vi "JT_Set_Monitor_Values.vi"(2 "Plot-Control":T1={"V2"=FALSE, "V5"=FALSE, "V1"=FALSE, "V9"=TRUE, "F"=TRUE, "C"=FALSE, "V4"=FALSE, "Dump"=0, "P3"=0.0, "P1"=0.0, "P2"=0.0, "P5"=18.434412358753207, "Box Temp"=18.434412358753207, "Pressure 1"=0, "Pressure 2"=0, "Pressure 3"=15, "Pressure 4"=13, "Setpoint"=0.0, "MC Heater Output"=0.0, "Still Heater Output"=0.0, "Sorb  Heater Output"=0.0, "Heater"=[], "Pressures"=[]} {"Pressure 4" items=["Time", "LI1CH1", "LI1CH2", "LI2CH1", "LI2CH2", "LI3CH1", "LI3CH2", "Field", "Temperature", "Temperature 2", "Temperatrue 3", "Nitrogen_Level", "Helium_Level", "Heater_LS370", "Sorb_Heater", "Still_Heater", "Capacity", "Loss", "Magnet_Temperature", "Lambda_Pressure", "Lambda_Needle_Valve", "LS370-CH1-T", "LS370-CH2-T", "LS370-CH3-T", "LS370-CH4-T", "LS370-TC-T", "LS370-CH1-R", "LS370-CH2-R", "LS370-CH3-R", "LS370-CH4-R", "LS370-TC-R", "LS372-CH1-T", "LS372-CH2-T", "LS372-CH3-T", "LS372-CH4-T", "LS372-CH5-T", "LS372-CH1-R", "LS372-CH2-R", "LS372-CH3-R", "LS372-CH4-R", "LS372-CH5-R", "Nada", "Keithley_Res", "Keithley_Current", "VTI_Heater", "VTI_Needle Valve", "LS340_Heater", "Keithley_6221_Amplitude", "Keithley_6221_Frequency", "Condense_Pressure", "Still_Pressure", "FP_Out_Pressure", "Dump_Pressure", "V1", "V2", "V4", "V5", "V9", "Forepump", "Compressor", "Keihtley_6221_Offset", "BoxTemp", "By", "Bz", "Phi", "heater-recond (%)", "Dewar Pressure "]; "Pressure 3" items=["Time", "LI1CH1", "LI1CH2", "LI2CH1", "LI2CH2", "LI3CH1", "LI3CH2", "Field", "Temperature", "Temperature 2", "Temperatrue 3", "Nitrogen_Level", "Helium_Level", "Heater_LS370", "Sorb_Heater", "Still_Heater", "Capacity", "Loss", "Magnet_Temperature", "Lambda_Pressure", "Lambda_Needle_Valve", "LS370-CH1-T", "LS370-CH2-T", "LS370-CH3-T", "LS370-CH4-T", "LS370-TC-T", "LS370-CH1-R", "LS370-CH2-R", "LS370-CH3-R", "LS370-CH4-R", "LS370-TC-R", "LS372-CH1-T", "LS372-CH2-T", "LS372-CH3-T", "LS372-CH4-T", "LS372-CH5-T", "LS372-CH1-R", "LS372-CH2-R", "LS372-CH3-R", "LS372-CH4-R", "LS372-CH5-R", "Nada", "Keithley_Res", "Keithley_Current", "VTI_Heater", "VTI_Needle Valve", "LS340_Heater", "Keithley_6221_Amplitude", "Keithley_6221_Frequency", "Condense_Pressure", "Still_Pressure", "FP_Out_Pressure", "Dump_Pressure", "V1", "V2", "V4", "V5", "V9", "Forepump", "Compressor", "Keihtley_6221_Offset", "BoxTemp", "By", "Bz", "Phi", "heater-recond (%)", "Dewar Pressure "]; "Pressure 2" items=["Time", "LI1CH1", "LI1CH2", "LI2CH1", "LI2CH2", "LI3CH1", "LI3CH2", "Field", "Temperature", "Temperature 2", "Temperatrue 3", "Nitrogen_Level", "Helium_Level", "Heater_LS370", "Sorb_Heater", "Still_Heater", "Capacity", "Loss", "Magnet_Temperature", "Lambda_Pressure", "Lambda_Needle_Valve", "LS370-CH1-T", "LS370-CH2-T", "LS370-CH3-T", "LS370-CH4-T", "LS370-TC-T", "LS370-CH1-R", "LS370-CH2-R", "LS370-CH3-R", "LS370-CH4-R", "LS370-TC-R", "LS372-CH1-T", "LS372-CH2-T", "LS372-CH3-T", "LS372-CH4-T", "LS372-CH5-T", "LS372-CH1-R", "LS372-CH2-R", "LS372-CH3-R", "LS372-CH4-R", "LS372-CH5-R", "Nada", "Keithley_Res", "Keithley_Current", "VTI_Heater", "VTI_Needle Valve", "LS340_Heater", "Keithley_6221_Amplitude", "Keithley_6221_Frequency", "Condense_Pressure", "Still_Pressure", "FP_Out_Pressure", "Dump_Pressure", "V1", "V2", "V4", "V5", "V9", "Forepump", "Compressor", "Keihtley_6221_Offset", "BoxTemp", "By", "Bz", "Phi", "heater-recond (%)", "Dewar Pressure "]; "Pressure 1" items=["Time", "LI1CH1", "LI1CH2", "LI2CH1", "LI2CH2", "LI3CH1", "LI3CH2", "Field", "Temperature", "Temperature 2", "Temperatrue 3", "Nitrogen_Level", "Helium_Level", "Heater_LS370", "Sorb_Heater", "Still_Heater", "Capacity", "Loss", "Magnet_Temperature", "Lambda_Pressure", "Lambda_Needle_Valve", "LS370-CH1-T", "LS370-CH2-T", "LS370-CH3-T", "LS370-CH4-T", "LS370-TC-T", "LS370-CH1-R", "LS370-CH2-R", "LS370-CH3-R", "LS370-CH4-R", "LS370-TC-R", "LS372-CH1-T", "LS372-CH2-T", "LS372-CH3-T", "LS372-CH4-T", "LS372-CH5-T", "LS372-CH1-R", "LS372-CH2-R", "LS372-CH3-R", "LS372-CH4-R", "LS372-CH5-R", "Nada", "Keithley_Res", "Keithley_Current", "VTI_Heater", "VTI_Needle Valve", "LS340_Heater", "Keithley_6221_Amplitude", "Keithley_6221_Frequency", "Condense_Pressure", "Still_Pressure", "FP_Out_Pressure", "Dump_Pressure", "V1", "V2", "V4", "V5", "V9", "Forepump", "Compressor", "Keihtley_6221_Offset", "BoxTemp", "By", "Bz", "Phi", "heater-recond (%)", "Dewar Pressure "]; "Dump" scale=0.0..100.0}, 3 "X-Axis (S)":i32, 4 "Measurement Time (s)":dbl format="%#_13g", 5 "System Monitor Variables (in)":T2) -> (0 "Cluster":T1={"V2"=FALSE, "V5"=FALSE, "V1"=FALSE, "V9"=TRUE, "F"=TRUE, "C"=FALSE, "V4"=FALSE, "Dump"=0, "P3"=0.0, "P1"=0.0, "P2"=0.0, "P5"=18.434412358753207, "Box Temp"=18.434412358753207, "Pressure 1"=0, "Pressure 2"=0, "Pressure 3"=15, "Pressure 4"=13, "Setpoint"=0.0, "MC Heater Output"=0.0, "Still Heater Output"=0.0, "Sorb  Heater Output"=0.0, "Heater"=[], "Pressures"=[]} {"Pressure 4" items=["Time", "LI1CH1", "LI1CH2", "LI2CH1", "LI2CH2", "LI3CH1", "LI3CH2", "Field", "Temperature", "Temperature 2", "Temperatrue 3", "Nitrogen_Level", "Helium_Level", "Heater_LS370", "Sorb_Heater", "Still_Heater", "Capacity", "Loss", "Magnet_Temperature", "Lambda_Pressure", "Lambda_Needle_Valve", "LS370-CH1-T", "LS370-CH2-T", "LS370-CH3-T", "LS370-CH4-T", "LS370-TC-T", "LS370-CH1-R", "LS370-CH2-R", "LS370-CH3-R", "LS370-CH4-R", "LS370-TC-R", "LS372-CH1-T", "LS372-CH2-T", "LS372-CH3-T", "LS372-CH4-T", "LS372-CH5-T", "LS372-CH1-R", "LS372-CH2-R", "LS372-CH3-R", "LS372-CH4-R", "LS372-CH5-R", "Nada", "Keithley_Res", "Keithley_Current", "VTI_Heater", "VTI_Needle Valve", "LS340_Heater", "Keithley_6221_Amplitude", "Keithley_6221_Frequency", "Condense_Pressure", "Still_Pressure", "FP_Out_Pressure", "Dump_Pressure", "V1", "V2", "V4", "V5", "V9", "Forepump", "Compressor", "Keihtley_6221_Offset", "BoxTemp", "By", "Bz", "Phi", "heater-recond (%)", "Dewar Pressure "]; "Pressure 3" items=["Time", "LI1CH1", "LI1CH2", "LI2CH1", "LI2CH2", "LI3CH1", "LI3CH2", "Field", "Temperature", "Temperature 2", "Temperatrue 3", "Nitrogen_Level", "Helium_Level", "Heater_LS370", "Sorb_Heater", "Still_Heater", "Capacity", "Loss", "Magnet_Temperature", "Lambda_Pressure", "Lambda_Needle_Valve", "LS370-CH1-T", "LS370-CH2-T", "LS370-CH3-T", "LS370-CH4-T", "LS370-TC-T", "LS370-CH1-R", "LS370-CH2-R", "LS370-CH3-R", "LS370-CH4-R", "LS370-TC-R", "LS372-CH1-T", "LS372-CH2-T", "LS372-CH3-T", "LS372-CH4-T", "LS372-CH5-T", "LS372-CH1-R", "LS372-CH2-R", "LS372-CH3-R", "LS372-CH4-R", "LS372-CH5-R", "Nada", "Keithley_Res", "Keithley_Current", "VTI_Heater", "VTI_Needle Valve", "LS340_Heater", "Keithley_6221_Amplitude", "Keithley_6221_Frequency", "Condense_Pressure", "Still_Pressure", "FP_Out_Pressure", "Dump_Pressure", "V1", "V2", "V4", "V5", "V9", "Forepump", "Compressor", "Keihtley_6221_Offset", "BoxTemp", "By", "Bz", "Phi", "heater-recond (%)", "Dewar Pressure "]; "Pressure 2" items=["Time", "LI1CH1", "LI1CH2", "LI2CH1", "LI2CH2", "LI3CH1", "LI3CH2", "Field", "Temperature", "Temperature 2", "Temperatrue 3", "Nitrogen_Level", "Helium_Level", "Heater_LS370", "Sorb_Heater", "Still_Heater", "Capacity", "Loss", "Magnet_Temperature", "Lambda_Pressure", "Lambda_Needle_Valve", "LS370-CH1-T", "LS370-CH2-T", "LS370-CH3-T", "LS370-CH4-T", "LS370-TC-T", "LS370-CH1-R", "LS370-CH2-R", "LS370-CH3-R", "LS370-CH4-R", "LS370-TC-R", "LS372-CH1-T", "LS372-CH2-T", "LS372-CH3-T", "LS372-CH4-T", "LS372-CH5-T", "LS372-CH1-R", "LS372-CH2-R", "LS372-CH3-R", "LS372-CH4-R", "LS372-CH5-R", "Nada", "Keithley_Res", "Keithley_Current", "VTI_Heater", "VTI_Needle Valve", "LS340_Heater", "Keithley_6221_Amplitude", "Keithley_6221_Frequency", "Condense_Pressure", "Still_Pressure", "FP_Out_Pressure", "Dump_Pressure", "V1", "V2", "V4", "V5", "V9", "Forepump", "Compressor", "Keihtley_6221_Offset", "BoxTemp", "By", "Bz", "Phi", "heater-recond (%)", "Dewar Pressure "]; "Pressure 1" items=["Time", "LI1CH1", "LI1CH2", "LI2CH1", "LI2CH2", "LI3CH1", "LI3CH2", "Field", "Temperature", "Temperature 2", "Temperatrue 3", "Nitrogen_Level", "Helium_Level", "Heater_LS370", "Sorb_Heater", "Still_Heater", "Capacity", "Loss", "Magnet_Temperature", "Lambda_Pressure", "Lambda_Needle_Valve", "LS370-CH1-T", "LS370-CH2-T", "LS370-CH3-T", "LS370-CH4-T", "LS370-TC-T", "LS370-CH1-R", "LS370-CH2-R", "LS370-CH3-R", "LS370-CH4-R", "LS370-TC-R", "LS372-CH1-T", "LS372-CH2-T", "LS372-CH3-T", "LS372-CH4-T", "LS372-CH5-T", "LS372-CH1-R", "LS372-CH2-R", "LS372-CH3-R", "LS372-CH4-R", "LS372-CH5-R", "Nada", "Keithley_Res", "Keithley_Current", "VTI_Heater", "VTI_Needle Valve", "LS340_Heater", "Keithley_6221_Amplitude", "Keithley_6221_Frequency", "Condense_Pressure", "Still_Pressure", "FP_Out_Pressure", "Dump_Pressure", "V1", "V2", "V4", "V5", "V9", "Forepump", "Compressor", "Keihtley_6221_Offset", "BoxTemp", "By", "Bz", "Phi", "heater-recond (%)", "Dewar Pressure "]; "Dump" scale=0.0..100.0}, 1 "System Monitor Variables (out)":T2)   [LabVIEW 2019]
uses:
  Global/Global Variables/System Monitor Cluster.ctl
  JT/JT-Status.ctl
  Global/Global Variables/Data_Display_global.vi
panel:
  # "Dill. unit"
  # "LN2\nTrap"
  # "12"
  # "15"
  # "Dill. unit"
  # "LN2\nTrap"
  # "12"
  # "15"
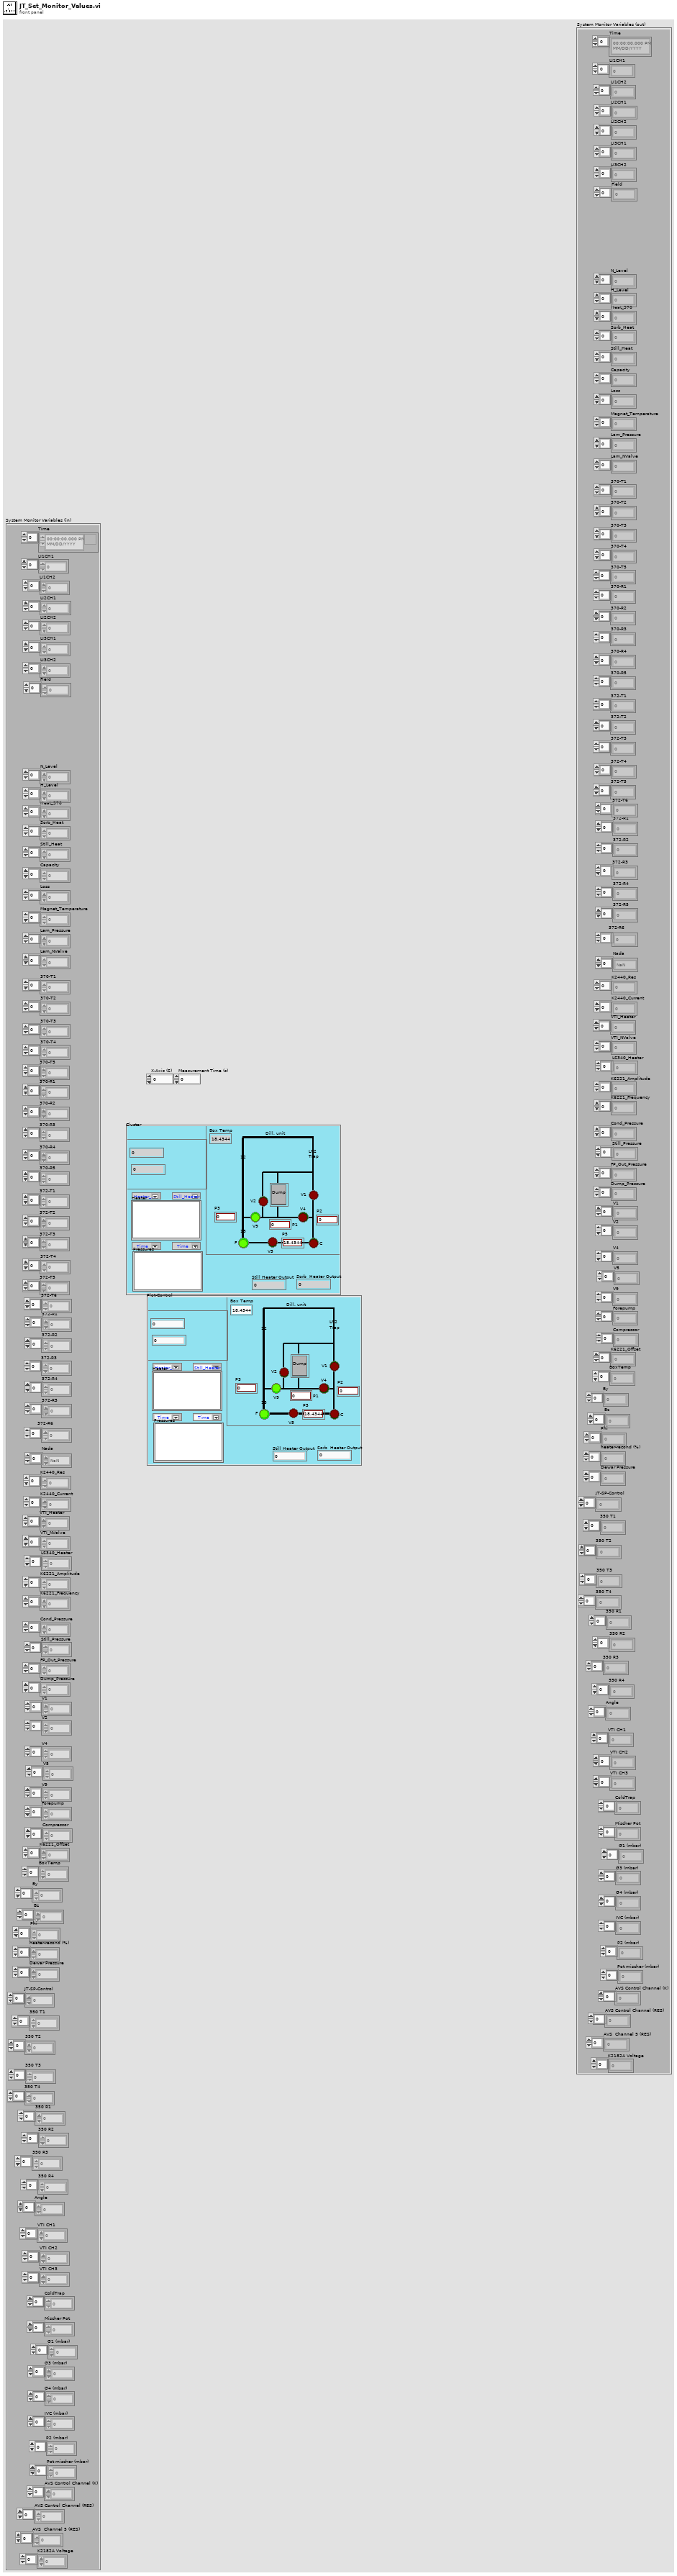
[diagram p1: front panel]
types:
  T1 = typedef "JT-Status.ctl" = cluster{"V2":bool, "V5":bool, "V1":bool, "V9":bool, "F":bool, "C":bool, "V4":bool, "Dump":u8, "P3":dbl, "P1":dbl, "P2":dbl, "P5":dbl, "Box Temp":dbl, "Pressure 1":i16, "Pressure 2":i16, "Pressure 3":i16, "Pressure 4":i16, "Setpoint":dbl, "MC Heater Output":dbl, "Still Heater Output":dbl, "Sorb  Heater Output":dbl, "Heater":dbl[][], "Pressures":dbl[][]}
  T2 = typedef "System Monitor Cluster.ctl" = cluster{"Time":timestamp[], "LI1CH1":dbl[], "LI1CH2":dbl[], "LI2CH1":dbl[], "LI2CH2":dbl[], "LI3CH1":dbl[], "LI3CH2":dbl[], "Field":dbl[], "N_Level":dbl[], "H_Level":dbl[], "Heat_370":dbl[], "Sorb_Heat":dbl[], "Still_Heat":dbl[], "Capacity":dbl[], "Loss":dbl[], "Magnet_Temperature":dbl[], "Lam_Pressure":dbl[], "Lam_NValve":dbl[], "370-T1":dbl[], "370-T2":dbl[], "370-T3":dbl[], "370-T4":dbl[], "370-T5":dbl[], "370-R1":dbl[], "370-R2":dbl[], "370-R3":dbl[], "370-R4":dbl[], "370-R5":dbl[], "372-T1":dbl[], "372-T2":dbl[], "372-T3":dbl[], "372-T4":dbl[], "372-T5":dbl[], "372-T6":dbl[], "372-R1":dbl[], "372-R2":dbl[], "372-R3":dbl[], "372-R4":dbl[], "372-R5":dbl[], "372-R6":dbl[], "Nada":dbl[], "K2440_Res":dbl[], "K2440_Current":dbl[], "VTI_Heater":dbl[], "VTI_NValve":dbl[], "LS340_Heater":dbl[], "K6221_Amplitude":dbl[], "K6221_Frequency":dbl[], "Cond_Pressure":dbl[], "Still_Pressure":dbl[], "FP_Out_Pressure":dbl[], "Dump_Pressure":dbl[], "V1":dbl[], "V2":dbl[], "V4":dbl[], "V5":dbl[], "V9":dbl[], "Forepump":dbl[], "Compressor":dbl[], "K6221_Offset":dbl[], "BoxTemp":dbl[], "By":dbl[], "Bz":dbl[], "Phi":dbl[], "heater-recond (%)":dbl[], "Dewar Pressure ":dbl[], "JT-SP-Control":dbl[], "350 T1":dbl[], "350 T2":dbl[], "350 T3":dbl[], "350 T4":dbl[], "350 R1":dbl[], "350 R2":dbl[], "350 R3":dbl[], "350 R4":dbl[], "Angle":dbl[], "VTI CH1":dbl[], "VTI CH2":dbl[], "VTI CH3":dbl[], "ColdTrap":dbl[], "Mischer Pot":dbl[], "G1 (mbar)":dbl[], "G3 (mbar) ":dbl[], "G4 (mbar)":dbl[], "IVC (mbar)":dbl[], "P2 (mbar) ":dbl[], "Pot mischer (mbar)":dbl[], "AVS Control Channel (K)":dbl[], "AVS Control Channel (RES)":dbl[], "AVS  Channel 5 (RES) ":dbl[], "K2182A Voltage":dbl[]}
  T3 = typedef "JT-Status-DD.ctl" = cluster{"V2":bool, "V5":bool, "V1":bool, "V9":bool, "F":bool, "C":bool, "V4":bool, "Dump":u8, "P3":dbl, "P1":dbl, "P2":dbl, "P5":dbl, "Box Temp":dbl}
  T4 = typedef "LS370_Status.ctl" = cluster{"Setpoint":dbl, "MC Heater Output":dbl, "Still Heater Output":dbl, "Sorb  Heater Output":dbl, "LS370 T1":dbl, "LS370 T2":dbl, "LS370 T3":dbl, "LS370 T4":dbl, "LS370 T5":dbl, "LS370 R1":dbl, "LS370 R2":dbl, "LS370 R3":dbl, "LS370 R4":dbl, "LS370 R5":dbl, "LS370 T6":dbl, "LS370 T7":dbl, "LS370 T8":dbl, "LS370 T9":dbl, "LS370 R6":dbl, "LS370 R7":dbl, "LS370 R8":dbl, "LS370 R9":dbl, "LS370 TC-T":dbl, "LS370 TC-R":dbl}
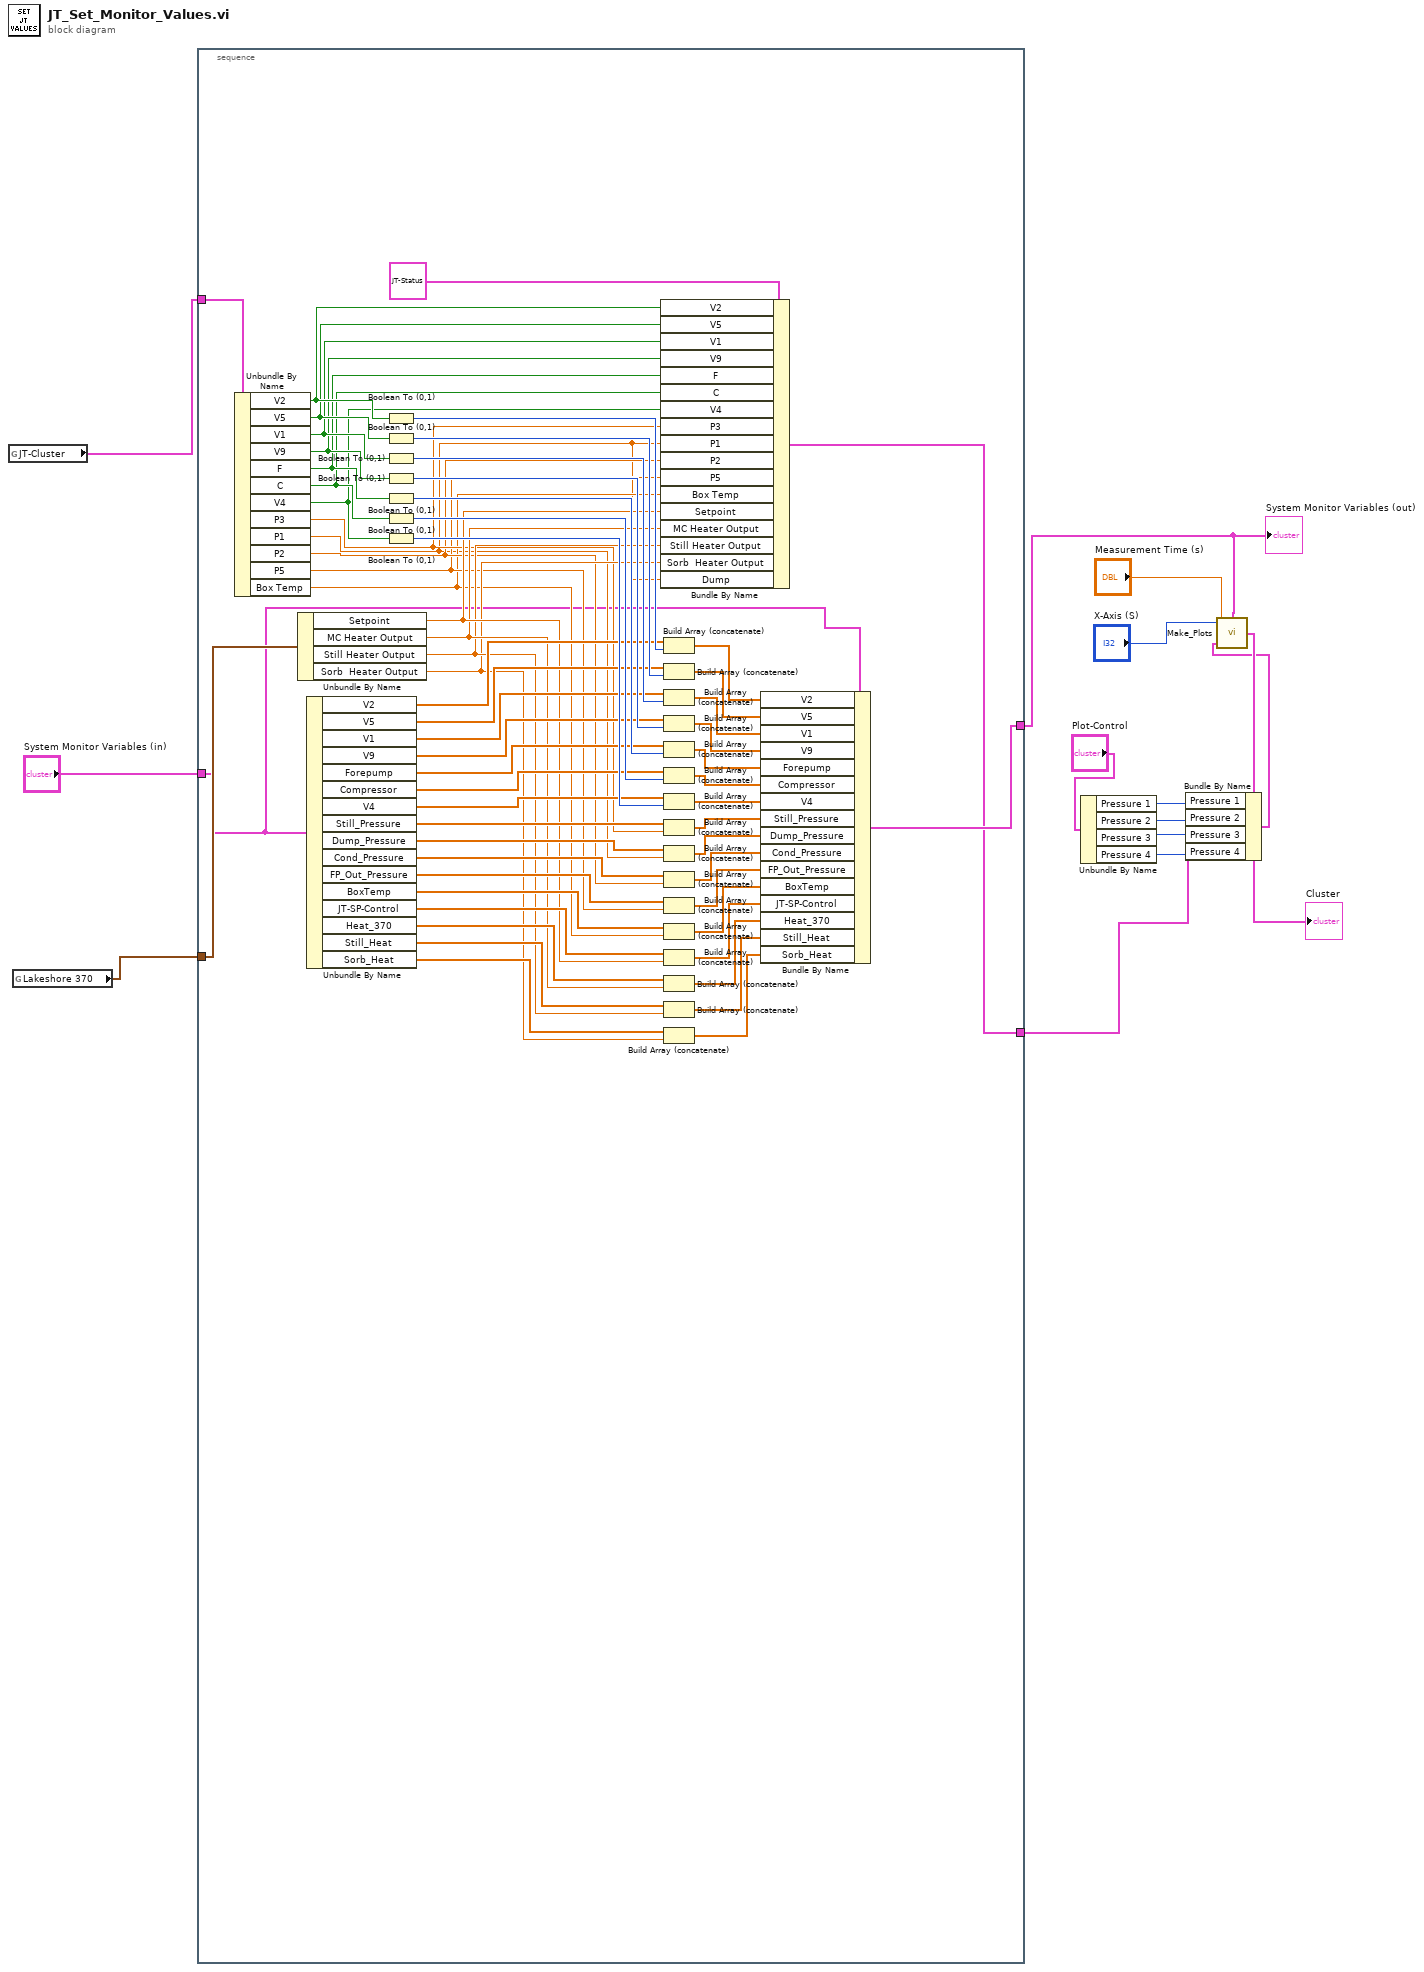
[diagram p0: block diagram]
diagram:
  n1 = global read "Data_Display_global.vi" "JT-Cluster"() -> (w13:T3)
  n2 = global read "Data_Display_global.vi" "Lakeshore 370"() -> (w12:T4)
  n3 = stacked-sequence {
    tunnel: "System Monitor Variables (in)" -> [w15]
    tunnel: [w35] -> w11
    tunnel: w13 -> [w75]
    tunnel: w12 -> [w34]
    tunnel: [w28] -> w5
    frame #0 {
      n4 = Unbundle By Name(w75) -> ("V2"=w27:bool, "V5"=w26:bool, "V1"=w25:bool, "V9"=w24:bool, "F"=w23:bool, "C"=w22:bool, "V4"=w21:bool, "P3"=w20:dbl, "P1"=w16:dbl, "P2"=w19:dbl, "P5"=w18:dbl, "Box Temp"=w17:dbl)
      n5 = Unbundle By Name(w34) -> ("Setpoint"=w32:dbl, "MC Heater Output"=w31:dbl, "Still Heater Output"=w30:dbl, "Sorb  Heater Output"=w29:dbl)
      n6 = Unbundle By Name(w15) -> ("V2"=w53:dbl[], "V5"=w54:dbl[], "V1"=w52:dbl[], "V9"=w56:dbl[], "Forepump"=w58:dbl[], "Compressor"=w57:dbl[], "V4"=w59:dbl[], "Still_Pressure"=w60:dbl[], "Dump_Pressure"=w61:dbl[], "Cond_Pressure"=w62:dbl[], "FP_Out_Pressure"=w63:dbl[], "BoxTemp"=w64:dbl[], "JT-SP-Control"=w65:dbl[], "Heat_370"=w66:dbl[], "Still_Heat"=w67:dbl[], "Sorb_Heat"=w68:dbl[])
      n7 = Boolean To (0,1)(Boolean=w27) -> (0, 1=w74:i16)
      n8 = Boolean To (0,1)(Boolean=w26) -> (0, 1=w73:i16)
      n9 = Boolean To (0,1)(Boolean=w25) -> (0, 1=w55:i16)
      n10 = Boolean To (0,1)(Boolean=w24) -> (0, 1=w72:i16)
      n11 = Boolean To (0,1)(Boolean=w23) -> (0, 1=w71:i16)
      n12 = Boolean To (0,1)(Boolean=w22) -> (0, 1=w70:i16)
      n13 = Boolean To (0,1)(Boolean=w21) -> (0, 1=w69:i16)
      n14 = Bundle By Name(cluster=T1 {"V2"=FALSE, "V5"=FALSE, "V1"=FALSE, "V9"=TRUE, "F"=TRUE, "C"=FALSE, "V4"=FALSE, "Dump"=0, "P3"=0.0, "P1"=0.0, "P2"=0.0, "P5"=18.434412358753207, "Box Temp"=18.434412358753207, "Pressure 1"=0, "Pressure 2"=0, "Pressure 3"=15, "Pressure 4"=13, "Setpoint"=0.0, "MC Heater Output"=0.0, "Still Heater Output"=0.0, "Sorb  Heater Output"=0.0, "Heater"=[], "Pressures"=[]} ("Cluster 2"), "V2"=w27, "V5"=w26, "V1"=w25, "V9"=w24, "F"=w23, "C"=w22, "V4"=w21, "P3"=w20, "P1"=w16, "P2"=w19, "P5"=w18, "Box Temp"=w17, "Setpoint"=w32, "MC Heater Output"=w31, "Still Heater Output"=w30, "Sorb  Heater Output"=w29, "Dump"=w16) -> (w28:T1)
      n15 = Build Array (concatenate)(w53, w74) -> (w51:dbl[])
      n16 = Build Array (concatenate)(w54, w73) -> (w50:dbl[])
      n17 = Build Array (concatenate)(w52, w55) -> (w49:dbl[])
      n18 = Build Array (concatenate)(w56, w72) -> (w48:dbl[])
      n19 = Build Array (concatenate)(w58, w71) -> (w47:dbl[])
      n20 = Build Array (concatenate)(w57, w70) -> (w46:dbl[])
      n21 = Build Array (concatenate)(w59, w69) -> (w45:dbl[])
      n22 = Build Array (concatenate)(w60, w20) -> (w44:dbl[])
      n23 = Build Array (concatenate)(w61, w16) -> (w43:dbl[])
      n24 = Build Array (concatenate)(w62, w19) -> (w42:dbl[])
      n25 = Build Array (concatenate)(w63, w18) -> (w41:dbl[])
      n26 = Build Array (concatenate)(w64, w17) -> (w40:dbl[])
      n27 = Build Array (concatenate)(w65, w32) -> (w39:dbl[])
      n28 = Build Array (concatenate)(w66, w31) -> (w38:dbl[])
      n29 = Build Array (concatenate)(w67, w30) -> (w37:dbl[])
      n30 = Build Array (concatenate)(w68, w29) -> (w36:dbl[])
      n31 = Bundle By Name(cluster=w15, "V2"=w51, "V5"=w50, "V1"=w49, "V9"=w48, "Forepump"=w47, "Compressor"=w46, "V4"=w45, "Still_Pressure"=w44, "Dump_Pressure"=w43, "Cond_Pressure"=w42, "FP_Out_Pressure"=w41, "BoxTemp"=w40, "JT-SP-Control"=w39, "Heat_370"=w38, "Still_Heat"=w37, "Sorb_Heat"=w36) -> (w35:T2)
    }
  }
  "System Monitor Variables (out)" <- w11
  n32 = Unbundle By Name("Plot-Control") -> ("Pressure 1"=w6:i16, "Pressure 2"=w4:i16, "Pressure 3"=w3:i16, "Pressure 4"=w2:i16)
  n33 = Bundle By Name(cluster=w5, "Pressure 1"=w6, "Pressure 2"=w4, "Pressure 3"=w3, "Pressure 4"=w2) -> (w1:T1)
  n34 = call "Make_Plots.vi"("System Monitor Variables"=w11, "JT-Cluster"=w1, "Measurement Time (s)"="Measurement Time (s)", "X-Axis (S)"="X-Axis (S)") -> ("JT-Cluster 2"=→"Cluster":T1)
